vi "Parse Connection List.vi"(8 "error in (no error)":errorcluster, 10 "connection list":string) -> (0 "error out":errorcluster, 2 "connections":T1[](array[typedef]))   [LabVIEW 2015, in "Route Manager.lvclass"]
uses:
  Route Manager.lvclass
  Connection.ctl
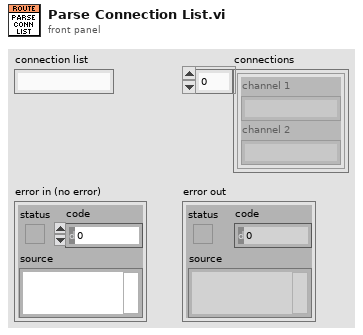
[diagram p1: front panel]
types:
  T1 = typedef "Route Manager.lvclass/Connection.ctl" = cluster{"channel 1":string, "channel 2":string}
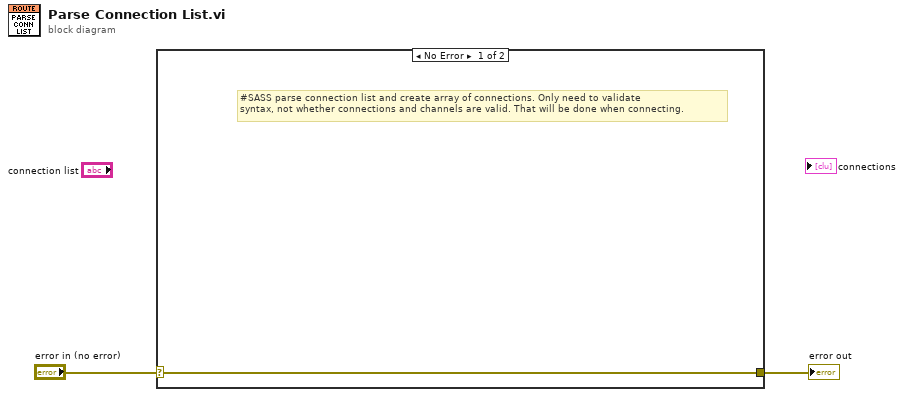
[diagram p0: block diagram]
diagram:
  n1 = case shown="No Error" "error in (no error)" {
    selector: "error in (no error)" -> [w3 w4]
    tunnel: [w3 w4] -> w1
    frame No Error {
      # "#SASS parse connection list and create array of connections. Only need to validate\nsyntax, not whether connections and channels are valid. That will be done when connecting."
    }
    frame Error {
    }
  }
  "error out" <- w1
